vi "INTERLOCK SETTING.vi"() -> ()   [LabVIEW 2017]
uses:
  <vilib>/addons/database/Connection.llb/DB Tools Open Connec (Path).vi
  <vilib>/addons/_office/excel.llb/Excel Get Data ([str]).vi
  <vilib>/addons/_office/excel.llb/Excel Easy Table (str).vi
  <vilib>/Utility/NIReport.llb/NI_report.lvclass
  <vilib>/addons/database/NI_Database_API.lvlib
  <vilib>/addons/_office/NI_ReportGenerationToolkit.lvlib
  <vilib>/Utility/NIReport.llb/Excel/NI_Excel.lvclass
panel:
  in  "RECIPE PATH":path
  in  "EXPORT RECIPE":bool
  in  "Import Recipe":bool
  in  "table":string[][](table)
  in  "EXIT":bool
  in  "SAVE":bool
  # "PARAMETERS VALUE"
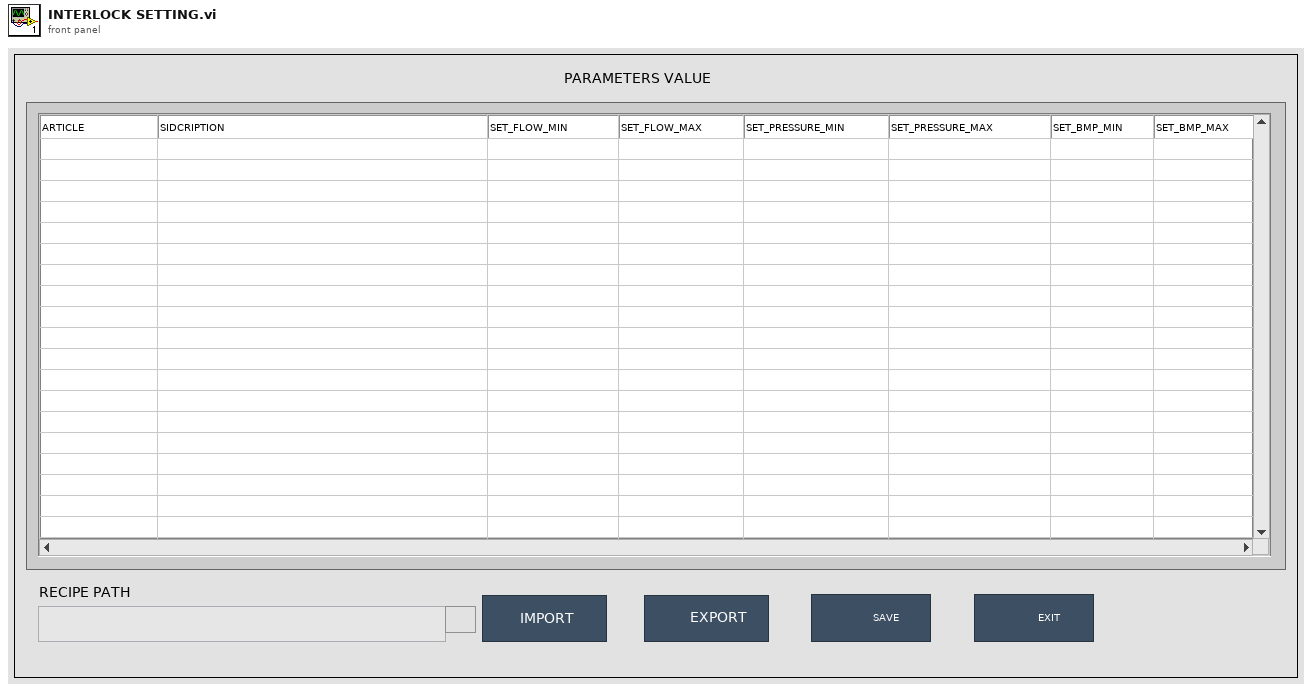
[diagram p1: front panel]
types:
  T1 = typedef "NI_Database_API.lvlib/Conn ObjectReference.ctl" = refnum<k1>
  T2 = enum16{"Standard Report", "HTML", "Word", "Excel"}
  T3 = enum16{"maximized", "minimized", "normal", "no change"}
  T4 = cluster{"table":string[], "table":string[], "table":string[], "table":string[], "table":string[], "table":string[], "table":string[], "table":string[]}
  T5 = enum32{"invalid app kind", "Development System", "Run Time System", "Student Edition", "Embedded LabVIEW", "Evaluation", "Custom"}
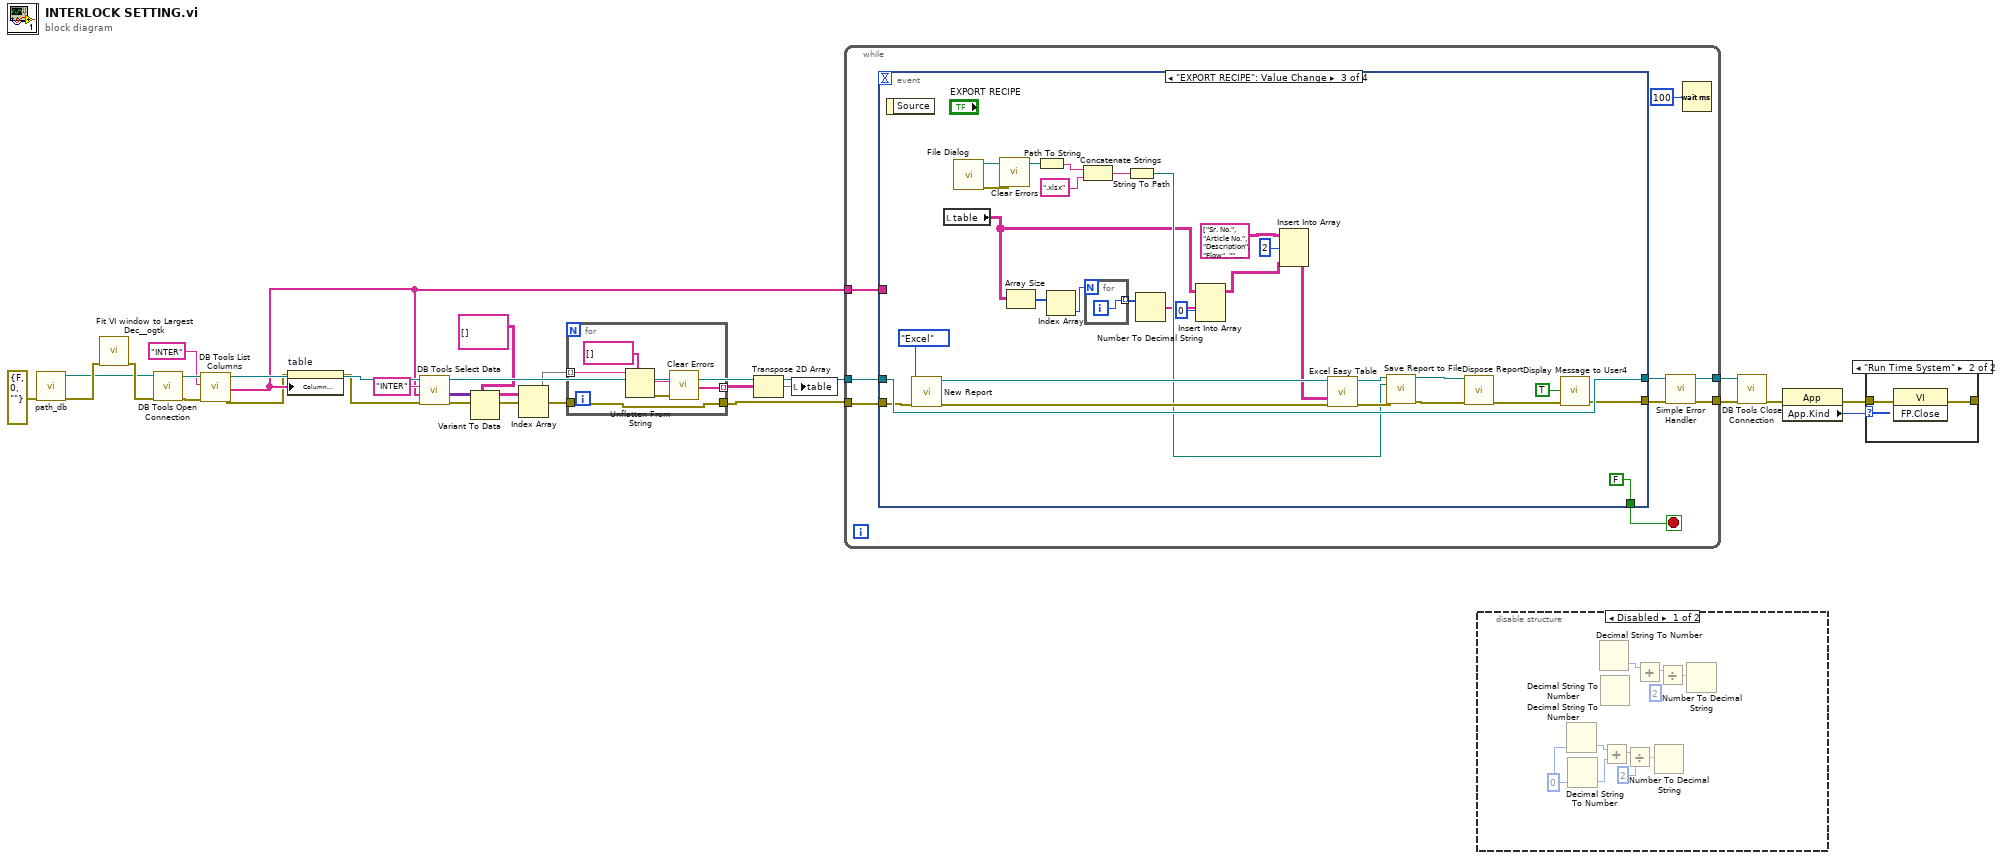
[diagram p0: block diagram]
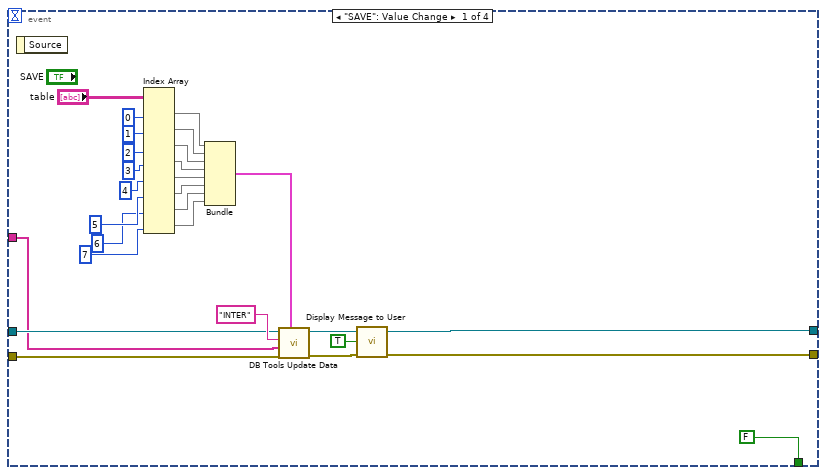
[diagram p4: hidden frame]
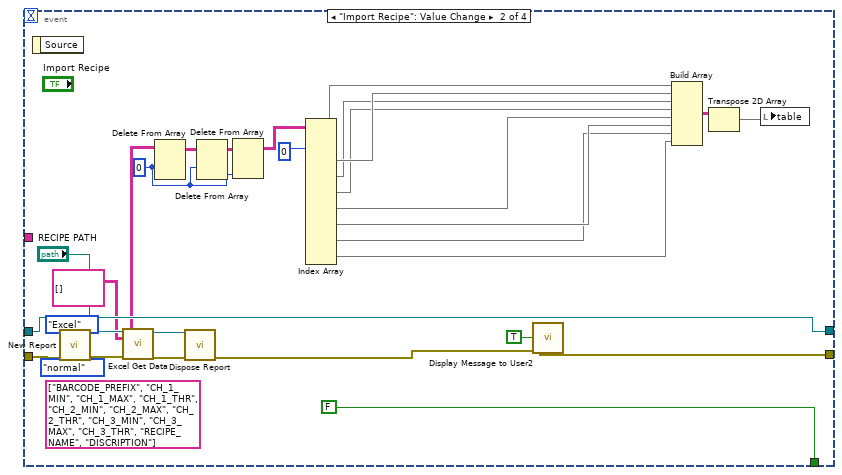
[diagram p5: hidden frame]
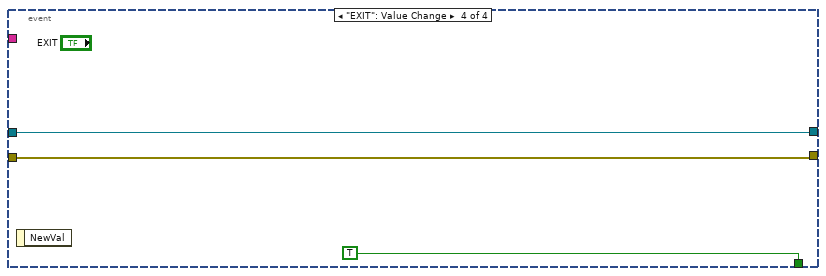
[diagram p6: hidden frame]
diagram:
  n1 = call "path_db.vi"("error in"=errorcluster {"status"=FALSE, "code"=0, "source"=""}) -> ("error out"=w11:errorcluster, "resulting string"=w1:path)  [unwired: 9 in]
  n2 = call <userlib>:"Fit VI window to Largest Dec__ogtk.vi"("error in (no error)"=w11) -> ("error out"=w10:errorcluster)  [unwired: 5 in, 1 out]
  n3 = call-poly <vilib>:"DB Tools Open Connection.vi"("error in (no error)"=w10, "connection information"=w1) -> ("error out"=w8:errorcluster, "connection reference"=w7:T1)  [unwired: 6 in]
  n4 = call <vilib>:"DB Tools List Columns.vi"("error in (no error)"=w8, "table"="INTER", "connection reference"=w7) -> ("error out"=w3:errorcluster, "columns"=w4:string[], "connection reference out"=w6:T1)  [unwired: 1 in, 1 out]
  n5 = property on="table" class="Tbl (strict)"(error in=w3, "Column Headers[]"=w4) -> (error out=w2:errorcluster)  [unwired: 1 in, 1 out]
  n6 = call <vilib>:"DB Tools Select Data.vi"("error in (no error)"=w2, "columns"=w4, "table"="INTER", "connection reference"=w6) -> ("error out"=w13:errorcluster, "data"=w18:variant[][], "connection reference out"=w21:T1)  [unwired: 2 in]
  n7 = Variant To Data(type=string[][] [], Variant=w18) -> (data=w17:string[][])  [unwired: 1 in, 1 out]
  n8 = Index Array(array=w17) -> (element=w15:string[])  [unwired: 2 in]
  n9 = for {
    tunnel: w15 -> [w30] mode=indexing
    tunnel: [w28] -> w14 mode=indexing
    tunnel: w13 -> [w27]
    tunnel: [w27] -> w12
    n10 = Unflatten From String(type=string[] [], binary string=w30) -> (value=w28:string[], error out=w31:errorcluster)  [unwired: 3 in, 1 out]
    n11 = call <vilib>:"Clear Errors.vi"("error in (no error)"=w31) -> ()  [unwired: 5 in, 2 out]
  }
  n12 = Transpose 2D Array(2D array=w14) -> (transposed array=w16:string[][])
  n13 = local write "table"(w16) -> ()
  n14 = while {
    tunnel: w12 -> [w38]
    tunnel: w21 -> [w37]
    tunnel: [w36] -> w26
    tunnel: [w34] -> w25
    tunnel: w4 -> [w32]
    stop <- w39 stop-if-true
    n15 = event shown="[2] \"EXPORT RECIPE\": Value Change" {
      selector: _ -> [_ _ _ _]
      dyn-events: _ -> [_ _ _ _]
      timeout: _ -> [_ _ _ _]
      tunnel: [FALSE FALSE FALSE TRUE] -> w39
      tunnel: w38 -> [w64 w84 w120 w127]
      tunnel: w37 -> [w63 w95 w124 w128]
      tunnel: [w62 w95 w124 w128] -> w36
      tunnel: [w42 w94 w123 w127] -> w35
      tunnel: w32 -> [w40 _ _ _]
      event "SAVE": Value Change {
        n16 = event-data() -> ()  [unwired: 1 in, 1 out]
        n17 = Index Array(array="table", index (col) #1=0 ("disabled index (col)"), index (col) #2=1 ("index (col)"), index (col) #3=2 ("index (col)"), index (col) #4=3 ("index (col)"), index (col) #5=4 ("index (col)"), index (col) #6=5 ("index (col)"), index (col) #7=6 ("index (col)"), index (col) #8=7 ("index (col)")) -> (element #1=w56:string[], element #2=w53:string[], element #3=w54:string[], element #4=w55:string[], element #5=w47:string[], element #6=w46:string[], element #7=w45:string[], element #8=w44:string[])  [unwired: 8 in]
        n18 = Bundle("table"=w56, "table"=w53, "table"=w54, "table"=w55, "table"=w47, "table"=w46, "table"=w45, "table"=w44) -> (w52:T4)  [unwired: 1 in]
        n19 = call <vilib>:"DB Tools Update Data.vi"("data"=w52, "error in (no error)"=w64, "columns"=w40, "table"="INTER", "connection reference"=w63) -> ("error out"=w43:errorcluster, "connection reference out"=w62:T1)  [unwired: 5 in]
        n20 = call "Display Message to User"("error in (no error)"=w43, "Enable"=TRUE) -> ("error out"=w42:errorcluster)  [unwired: 8 in, 1 out]
      }
      event "Import Recipe": Value Change {
        w80 = 0 ("index (row)")
        (unwired) string[] ["BARCODE_PREFIX", "CH_1_MIN", "CH_1_MAX", "CH_1_THR", "CH_2_MIN", "CH_2_MAX", "CH_2_THR", "CH_3_MIN", "CH_3_MAX", "CH_3_THR", "RECIPE_NAME", "DISCRIPTION"]
        n21 = event-data() -> ()  [unwired: 1 in, 1 out]
        n22 = call <vilib>:"New Report.vi"("window state (normal)"=T3."normal", "report type"=T2."Excel", "template (empty)"="RECIPE PATH", "error in (no error)"=w84) -> ("report out"=w87:refnum<class "NI_report.lvclass">, "error out"=w88:errorcluster)  [unwired: 10 in]
        n23 = call-poly <vilib>:"Excel Get Data.vi"("report in"=w87, "data type"=string[][] [], "error in (no error)"=w88) -> ("report out"=w89:refnum<class "NI_report.lvclass">, "data"=w67:string[][], "error out"=w90:errorcluster)  [unwired: 10 in]
        n24 = Delete From Array(array=w67, index (row)=w80) -> (array with subset deleted=w82:string[][])  [unwired: 2 in, 1 out]
        n25 = call-dynamic "Dispose Report.vi"("report in"=w89, "error in (no error)"=w90) -> ("error out"=w83:errorcluster)  [unwired: 13 in]
        n26 = Delete From Array(array=w82, index (row)=w80) -> (array with subset deleted=w81:string[][])  [unwired: 2 in, 1 out]
        n27 = Delete From Array(array=w81, index (col)=w80) -> (array with subset deleted=w79:string[][])  [unwired: 2 in, 1 out]
        n28 = Index Array(array=w79, index (col) #1=0 ("disabled index (col)")) -> (element #1=w77:string[], element #2=w76:string[], element #3=w73:string[], element #4=w72:string[], element #5=w71:string[], element #6=w70:string[], element #7=w69:string[], element #8=w68:string[])  [unwired: 15 in]
        n29 = call "Display Message to User2"("error in (no error)"=w83, "Enable"=TRUE) -> ("error out"=w94:errorcluster)  [unwired: 8 in, 1 out]
        n30 = Build Array(w77, w76, w73, w72, w71, w70, w69, w68) -> (w75:string[][])
        n31 = Transpose 2D Array(2D array=w75) -> (transposed array=w74:string[][])
        n32 = local write "table"(w74) -> ()
      }
      event "EXPORT RECIPE": Value Change {
        n33 = event-data() -> ()  [unwired: 1 in, 1 out]
        n34 = call <vilib>:"New Report.vi"("report type"=T2."Excel", "error in (no error)"=w120) -> ("report out"=w112:refnum<class "NI_report.lvclass">, "error out"=w113:errorcluster)  [unwired: 12 in]
        n35 = local read "table"() -> (w98:string[][])
        n36 = call "File Dialog"() -> ("selected path"=w114:path, "error out"=w118:errorcluster)  [unwired: 12 in, 2 out]
        n37 = call <vilib>:"Clear Errors.vi"("error in (no error)"=w118) -> ()  [unwired: 5 in, 2 out]
        n38 = Array Size(array=w98) -> (size(s)=w106:i32[])
        n39 = Path To String(path=w114) -> (string=w115:string)
        n40 = Index Array(array=w106) -> (element=w105:i32)  [unwired: 1 in]
        n41 = Concatenate Strings(w115, ".xlsx" ("string")) -> (w117:string)
        n42 = for {
          N: w105 -> [_]
          tunnel: [w126] -> w104 mode=indexing
          i -> [w126]
        }
        n43 = String To Path(string=w117) -> (path=w107:path)
        n44 = Number To Decimal String(number=w104) -> (decimal integer string=w103:string[])  [unwired: 1 in]
        n45 = Insert Into Array(array=w98, index (col)=0 ("disabled index (col)"), new element=w103) -> (w102:string[][])  [unwired: 1 in]
        n46 = Insert Into Array(array=string[][] [["Sr. No.", "Article No.", "Description", "Flow", "", "Pressure", "", "BPM", ""], ["", "", "", "Min", "Max", "Min", "Max", "Min", "Max"]] ("appended array"), index (row)=2, new element=w102) -> (w97:string[][])  [unwired: 1 in]
        n47 = call-poly <vilib>:"Excel Easy Table.vi"("report in"=w112, "text data"=w97, "error in (no error)"=w113) -> ("report out"=w109:refnum<class "NI_report.lvclass">, "error out"=w111:errorcluster)  [unwired: 8 in, 3 out]
        n48 = call-dynamic "Save Report to File.vi"("report in"=w109, "report file path"=w107, "error in (no error)"=w111) -> ("report out"=w108:refnum<class "NI_report.lvclass">, "error out"=w110:errorcluster)  [unwired: 11 in]
        n49 = call-dynamic "Dispose Report.vi"("report in"=w108, "error in (no error)"=w110) -> ("error out"=w119:errorcluster)  [unwired: 13 in]
        n50 = call "Display Message to User4"("error in (no error)"=w119, "Enable"=TRUE) -> ("error out"=w123:errorcluster)  [unwired: 8 in, 1 out]
      }
      event "EXIT": Value Change {
        n51 = event-data() -> ()  [unwired: 1 in, 1 out]
      }
    }
    n52 = call <vilib>:"Simple Error Handler.vi"("error in (no error)"=w35) -> ("error out"=w34:errorcluster)  [unwired: 4 in, 4 out]
    n53 = Wait (ms)(milliseconds to wait=u32 100) -> ()  [unwired: 1 out]
  }
  n54 = disable-structure shown="Disabled" {
    frame Disabled {
      (unwired) 2
      w133 = u64 0 ("default (0 I32)")
      n55 = Decimal String To Number(default (0L)=w133) -> (number=w135:u64)  [unwired: 2 in, 1 out]
      n56 = Decimal String To Number(default (0L)=w133) -> (number=w136:u64)  [unwired: 2 in, 1 out]
      n57 = Decimal String To Number() -> (number=w132:i32)  [unwired: 3 in, 1 out]
      n58 = Decimal String To Number() -> ()  [unwired: 3 in, 2 out]
      n59 = Add(x=w135, y=w136) -> (x+y=w137:u64)
      n60 = Divide(x=w137, y=2) -> (x/y=w138:dbl)
      n61 = Add(x=w132) -> (x+y=w131:i32)  [unwired: 1 in]
      n62 = Number To Decimal String(number=w138) -> ()  [unwired: 1 in, 1 out]
      n63 = Divide(x=w131) -> (x/y=w130:dbl)  [unwired: 1 in]
      n64 = Number To Decimal String(number=w130) -> ()  [unwired: 1 in, 1 out]
    }
    frame Enabled {
    }
  }
  n65 = call <vilib>:"DB Tools Close Connection.vi"("error in (no error)"=w25, "connection reference"=w26) -> ("error out"=w22:errorcluster)  [unwired: 5 in]
  n66 = property class="App"(error in=w22) -> (error out=w23:errorcluster, "App.Kind"=w24:T5)  [unwired: 1 in, 1 out]
  n67 = case shown="\"Run Time System\"" w24 {
    tunnel: w23 -> [w139 w141]
    tunnel: [w139 w140] -> _
    frame Default {
    }
    frame "Run Time System" {
      n68 = invoke class="VI" method="FP.Close"(error in=w141) -> (error out=w140:errorcluster)  [unwired: 2 in, 2 out]
    }
  }
